vi "Read Response destination.vi"(8 "error in (no error)":errorcluster, 11 "Reward_Condition in":refnum<class "Reward_Condition.lvclass">) -> (0 "error out":errorcluster, 2 "Response destination":T1(ring), 3 "Reward_Condition out":refnum<class "Reward_Condition.lvclass">)   [LabVIEW 2018, in "Tracker.lvlib" / "Reward_Condition.lvclass"]
uses:
  Reward_Condition.lvclass
  Reward_Condition.lvclass/Reward_Condition.ctl
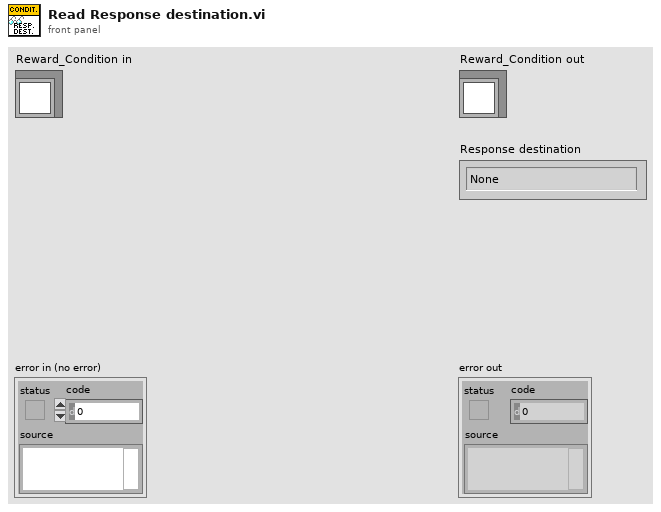
[diagram p1: front panel]
types:
  T1 = enum16{"None", "Port 1", "Port 2", "Port 3", "Port 4"}
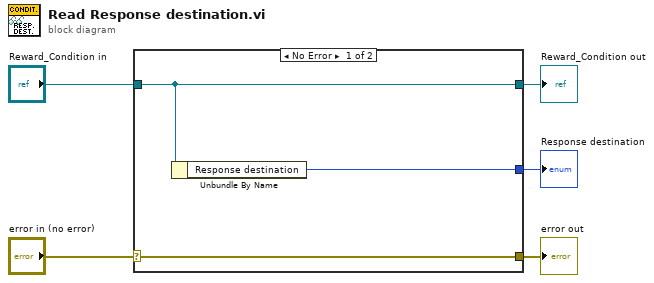
[diagram p0: block diagram]
diagram:
  n1 = case shown="No Error" "error in (no error)" {
    selector: "error in (no error)" -> [w8 w9]
    tunnel: [w8 w9] -> w4
    tunnel: [w7 w10] -> w2
    tunnel: "Reward_Condition in" -> [w7 w10]
    tunnel: [w6 _] -> w1
    frame No Error {
      n2 = Unbundle By Name(w7) -> ("Response destination"=w6:T1)
    }
    frame Error {
    }
  }
  "error out" <- w4
  "Reward_Condition out" <- w2
  "Response destination" <- w1
